vi "Error handler.vi"(10 "error in":errorcluster, 11 "Error reason":string) -> ()   [LabVIEW 2016]
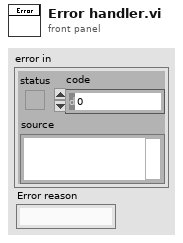
[diagram p1: front panel]
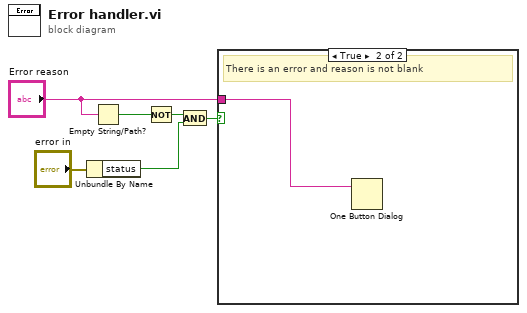
[diagram p0: block diagram]
diagram:
  n1 = Unbundle By Name("error in") -> ("status"=w1:bool)
  n2 = Empty String/Path?(string/path="Error reason") -> (empty?=w4:bool)
  n3 = Not(x=w4) -> (.not. x?=w3:bool)
  n4 = And(x=w3, y=w1) -> (x .and. y?=w2:bool)
  n5 = case shown="True" w2 {
    tunnel: "Error reason" -> [_ w7]
    frame False {
      # "Display nothin."
    }
    frame True {
      # "There is an error and reason is not blank"
      n6 = One Button Dialog(message=w7) -> ()  [unwired: 1 in, 1 out]
    }
  }
